vi "niScope Auto Setup.vi"(0 "instrument handle":refnum<k15>, 11 "error in":errorcluster) -> (4 "instrument handle out":refnum<k15>, 15 "error out":errorcluster)   [LabVIEW 2011]
doc: "Automatically configures the digitizer."
uses:
  niScope_32.dll
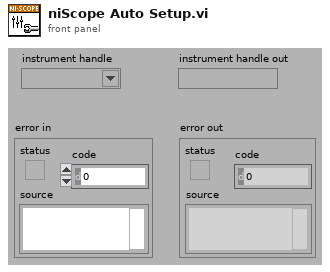
[diagram p1: front panel]
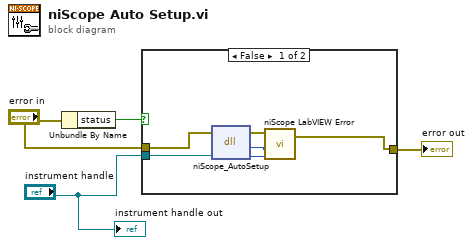
[diagram p0: block diagram]
diagram:
  n1 = Unbundle By Name("error in") -> ("status"=w3:bool)
  n2 = case shown="False" w3 {
    tunnel: "error in" -> [w6 w10]
    tunnel: [w5 w10] -> w2
    tunnel: "instrument handle" -> [w9 _]
    frame False {
      n3 = dll-call lib="niScope_*.*" fn="niScope_AutoSetup"("instrument handle"=w9) -> ("status"=w8:i32, "instrument handle"=w7:u32)  [unwired: 3 in, 2 out]
      n4 = call <instrlib>:"niScope LabVIEW Error.vi"("instrument handle"=w7, "niScope error code (0)"=w8, "error in (no error)"=w6) -> ("error out"=w5:errorcluster)  [unwired: 2 in]
    }
    frame True {
    }
  }
  "error out" <- w2
  "instrument handle out" <- "instrument handle"
